vi "Initialize.vi"(4 "X column":i32, 6 "Bin":dbl, 7 "Number of columns":i32, 8 "error in (no error)":errorcluster, 9 "Number of rows":i32, 10 "Start":dbl, 11 "Bin Average in":refnum<class "Bin Average.lvclass">) -> (0 "error out":errorcluster, 3 "Bin Average out":refnum<class "Bin Average.lvclass">)   [LabVIEW 2016, in "Bin Average.lvclass"]
uses:
  Bin Average.lvclass
  Bin Average.lvclass/Bin Average.ctl
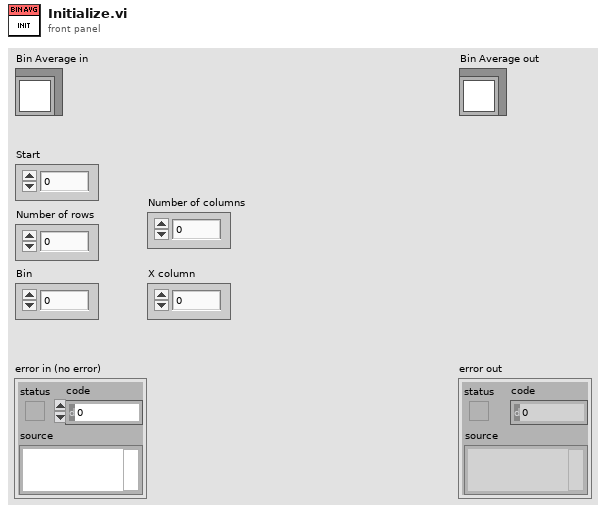
[diagram p1: front panel]
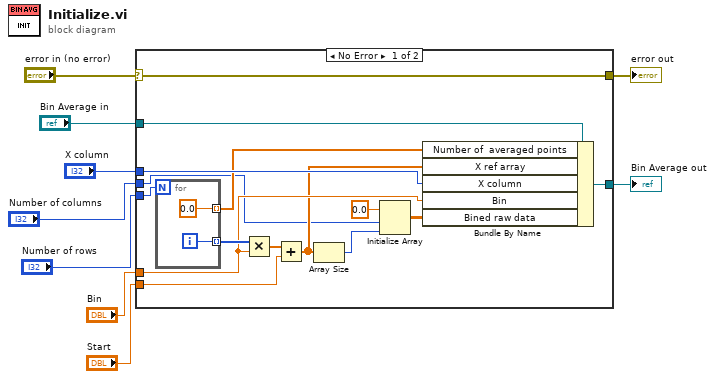
[diagram p0: block diagram]
diagram:
  n1 = case shown="No Error" "error in (no error)" {
    selector: "error in (no error)" -> [w23 w28]
    tunnel: [w23 w28] -> w8
    tunnel: [w18 w27] -> w6
    tunnel: "Bin Average in" -> [w24 w27]
    tunnel: "Number of rows" -> [w22 _]
    tunnel: "Start" -> [w19 _]
    tunnel: "Bin" -> [w15 _]
    tunnel: "X column" -> [w17 _]
    tunnel: "Number of columns" -> [w10 _]
    frame No Error {
      n2 = for {
        N: w22 -> [_]
        tunnel: [w26] -> w21 mode=indexing
        tunnel: [0.0] -> w16 mode=indexing
        i -> [w26]
      }
      n3 = Multiply(x=w21, y=w15) -> (x*y=w20:dbl[])
      n4 = Add(x=w20, y=w19) -> (x+y=w12:dbl[])
      n5 = Array Size(array=w12) -> (size(s)=w13:i32)
      n6 = Initialize Array(0.0, w10, w13) -> (w11:dbl[][])
      n7 = Bundle By Name(cluster=w24, "Number of  averaged points"=w16, "X ref array"=w12, "X column"=w17, "Bin"=w15, "Bined raw data"=w11) -> (w18:refnum<class "Bin Average.lvclass">)
    }
    frame Error {
    }
  }
  "error out" <- w8
  "Bin Average out" <- w6
